vi "add module to engine.vi"(8 "error in":errorcluster, 10 "module ID":string, 11 "engine configuration in":refnum<class "engine configuration.lvclass">) -> (0 "error out":errorcluster, 3 "engine configuration out":refnum<class "engine configuration.lvclass">)   [LabVIEW 2013, in "engine configuration.lvclass"]
uses:
  engine configuration.lvclass
  engine configuration.lvclass/engine configuration.ctl
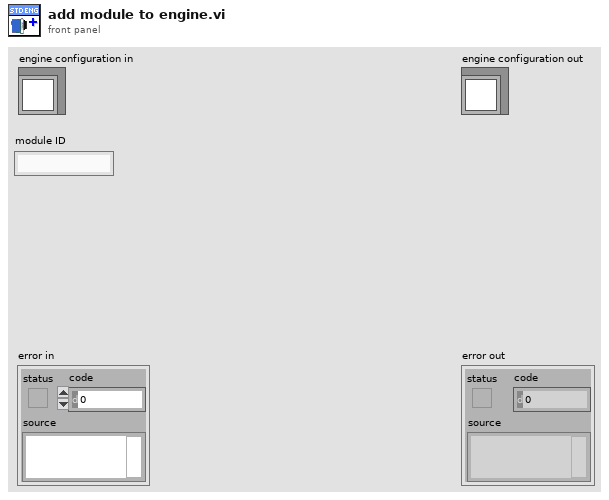
[diagram p1: front panel]
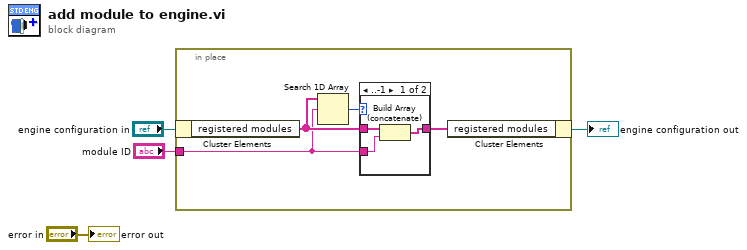
[diagram p0: block diagram]
diagram:
  n1 = in-place {
    in-place-border: "module ID" -> [w5]
    n2 = in-place-cluster #1("engine configuration in") -> ("registered modules"=w6:string[])
    n3 = Search 1D Array(1D array=w6, element=w5) -> (index of element=w8:i32)  [unwired: 1 in]
    n4 = case shown="..-1" w8 {
      tunnel: [w11 w12] -> w7
      tunnel: w6 -> [w10 w12]
      tunnel: w5 -> [w9 _]
      frame ..-1 {
        n5 = Build Array (concatenate)(w10, w9) -> (w11:string[])
      }
      frame 0.. {
      }
    }
    n6 = in-place-cluster #1("registered modules"=w7) -> (→"engine configuration out":refnum<class "engine configuration.lvclass">)
  }
  "error out" <- "error in"
